vi "Configure Module.vi"(5 "Worktable Mode":T1, 7 "Config Manager":refnum<class "Config Manager Class.lvclass">, 8 "error in":errorcluster, 11 "WorkTable in":refnum<class "WorkTable Class.lvclass">) -> (0 "error out":errorcluster, 3 "WorkTable out":refnum<class "WorkTable Class.lvclass">)   [LabVIEW 2011, in "WorkTable Class.lvclass"]
uses:
  WorkTable Class.lvclass
  Config Manager Class/Config Manager Class.lvclass
  Type Definitions/Worktable_Mode.ctl
  Config Manager Class/Type Definitions/Part Type.ctl
  Type Definitions/Worktable_Module Slot.ctl
  Utils/Type Definitions/Position_Orientation.ctl
  Vec3d Class/Vec3d Class.lvclass
  Orient3d Class/Orient3d Class.lvclass
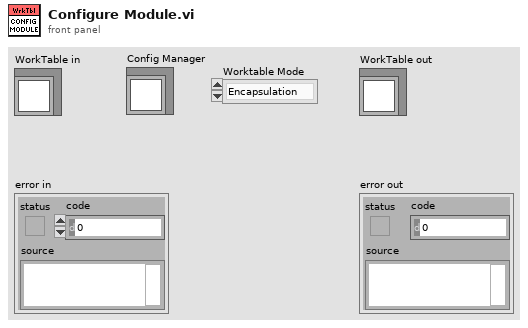
[diagram p1: front panel]
types:
  T1 = typedef "Worktable_Mode.ctl" = enum16{"Encapsulation", "Gluing"}
  T2 = typedef "Part Type.ctl" = enum16{"BBM", "HDI", "BARE HDI", "GLUERESERVOIR", "STAMP_1", "STAMP_2", "STAMP_3", "STAMP_4", "STAMP_5", "WEIGHT_1", "WEIGHT_2", "WEIGHT_3", "WEIGHT_4", "WEIGHT_5", "WEIGHT_6", "WEIGHT_7", "WEIGHT_8", "PICKER_TOOL", "GRABER_TOOL"}
  T3 = typedef "Worktable_Module Slot.ctl" = cluster{"Slot State":enum16{"Empty", "Bare HDI", "Unglued", "Stamped", "PartOnTop", "Weighted", "Unpotted", "Potted"}, "BBM Type":enum16{"None", "BBM", "GlassSlide"}, "HDI Type":enum16{"None", "HDI", "Polyimide"}, "Vacuum Channel":u8, "Location/Orientation BBM":T4, "Location/Orientation HDI":T4, "S/N":string}
  T4 = typedef "Position_Orientation.ctl" = cluster{"Center":refnum<class "Vec3d Class.lvclass">, "Orientation":refnum<class "Orient3d Class.lvclass">}
  T5 = enum16{"Empty", "Bare HDI", "Unglued", "Stamped", "PartOnTop", "Weighted", "Unpotted", "Potted"}
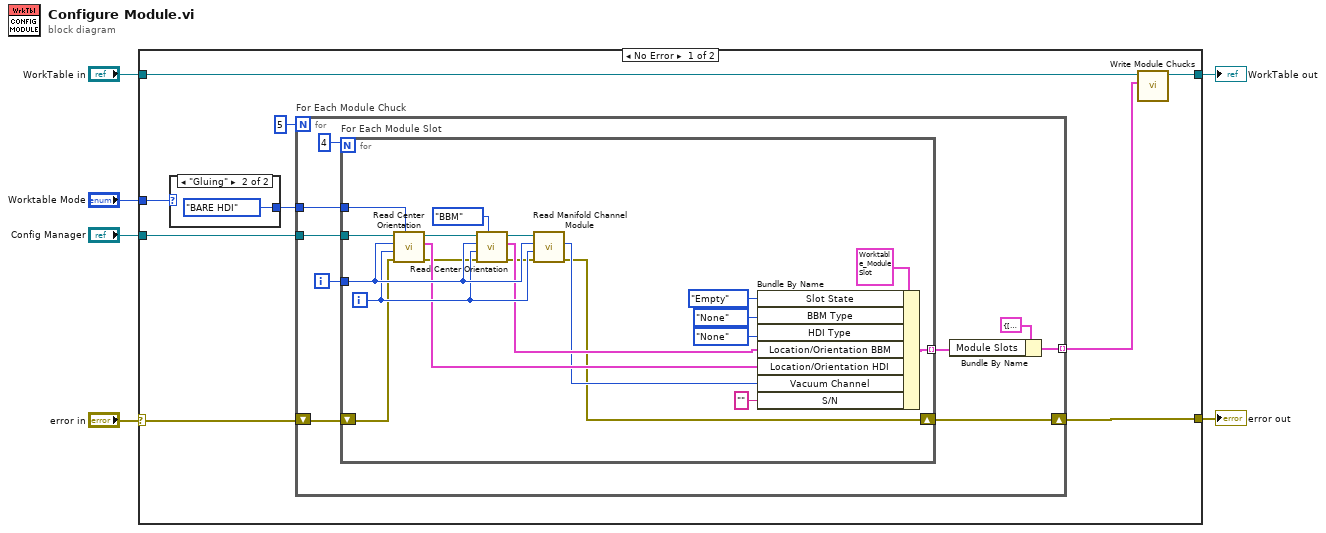
[diagram p0: block diagram]
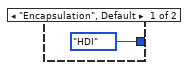
[diagram p2: hidden frame]
diagram:
  n1 = case shown="No Error" "error in" {
    selector: "error in" -> [w10 w48]
    tunnel: [w9 w48] -> w5
    tunnel: "WorkTable in" -> [w13 w47]
    tunnel: [w14 w47] -> w3
    tunnel: "Config Manager" -> [w11 _]
    tunnel: "Worktable Mode" -> [w8 _]
    frame No Error {
      n2 = case shown="\"Gluing\"" w8 {
        tunnel: [Part_Type."HDI" ("Part Type") Part_Type."BARE HDI" ("Part Type")] -> w7
        frame "Encapsulation", Default {
        }
        frame "Gluing" {
        }
      }
      n3 = for "For Each Module Chuck" {
        N: 5 -> [_]
        tunnel: [w23] -> w12 mode=indexing
        shift-right: [w19] -> w9
        shift-left: w10 -> [w20]
        tunnel: w11 -> [w22]
        tunnel: w7 -> [w18]
        i -> [w21]
        n4 = for "For Each Module Slot" {
          N: 4 ("dimension size") -> [_]
          tunnel: [w46] -> w24 mode=indexing
          tunnel: w21 -> [w37]
          shift-right: [w29] -> w19
          shift-left: w20 -> [w32]
          tunnel: w22 -> [w41]
          tunnel: w18 -> [w28]
          i -> [w36]
          n5 = call "Read Center Orientation.vi"("Part Type"=w28, "error in"=w32, "slot"=w36, "chuck"=w37, "Config Manager in"=w41) -> ("error out"=w31:errorcluster, "Location/Orientation"=w35:T4, "Config Manager out"=w40:refnum<class "Config Manager Class.lvclass">)  [unwired: 4 in]
          n6 = call "Read Center Orientation.vi"("Part Type"=Part_Type."BBM", "error in"=w31, "slot"=w36, "chuck"=w37, "Config Manager in"=w40) -> ("error out"=w30:errorcluster, "Location/Orientation"=w34:T4, "Config Manager out"=w39:refnum<class "Config Manager Class.lvclass">)  [unwired: 4 in]
          n7 = call "Read Manifold Channel Module.vi"("error in"=w30, "Slot"=w36, "Chuck"=w37, "Config Manager in"=w39) -> ("error out"=w29:errorcluster, "Channel"=w33:i32)  [unwired: 5 in, 1 out]
          n8 = Bundle By Name(cluster=T3 {"Slot State"=enum."Empty", "BBM Type"=enum."BBM", "HDI Type"=enum."HDI", "Vacuum Channel"=0, "Location/Orientation BBM"={"Center"=refnum, "Orientation"=refnum}, "Location/Orientation HDI"={"Center"=refnum, "Orientation"=refnum}, "S/N"=""} ("element"), "Slot State"=T5."Empty", "BBM Type"=enum16{"None", "BBM", "GlassSlide"}."None", "HDI Type"=enum16{"None", "HDI", "Polyimide"}."None", "Location/Orientation BBM"=w34, "Location/Orientation HDI"=w35, "Vacuum Channel"=w33, "S/N"="") -> (w46:T3)
        }
        n9 = Bundle By Name(cluster=cluster{"Module Slots":T3[]} {"Module Slots"=[{"Slot State"=enum."Empty", "BBM Type"=enum."BBM", "HDI Type"=enum."HDI", "Vacuum Channel"=0, "Location/Orientation BBM"={"Center"=refnum, "Orientation"=refnum}, "Location/Orientation HDI"={"Center"=refnum, "Orientation"=refnum}, "S/N"=""}]} ("Module Chuck"), "Module Slots"=w24) -> (w23:cluster{"Module Slots":T3[]})
      }
      n10 = call-dynamic "Write Module Chucks.vi"("Module Chucks"=w12, "WorkTable in"=w13) -> ("WorkTable out"=w14:refnum<class "WorkTable Class.lvclass">)  [unwired: 8 in, 1 out]
    }
    frame Error {
    }
  }
  "WorkTable out" <- w3
  "error out" <- w5
